vi "cwlaserShutterFromWavelength.vi"(0 "wavelength (nm)":dbl) -> (1 "shutter":i32, 2 "found":bool)   [LabVIEW 2017]
uses:
  globalDevices.vi
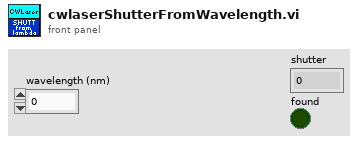
[diagram p1: front panel]
types:
  T1 = cluster{"serialPort":refnum<visa-resource-name>, "error":errorcluster, "power (mW)":dbl, "wavelength (nm)":dbl, "type":string, "shutter":i32}[]
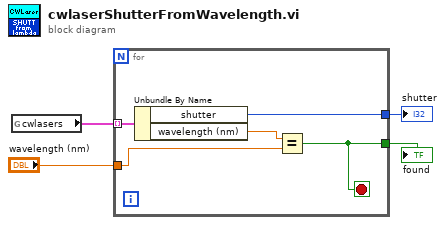
[diagram p0: block diagram]
diagram:
  n1 = global read "globalDevices.vi" "cwlasers"() -> (w4:T1)
  n2 = for {
    tunnel: w4 -> [w9] mode=indexing
    tunnel: "wavelength (nm)" -> [w7]
    tunnel: [w6] -> w2
    tunnel: [w5] -> w1
    stop <- w5 stop-if-true
    n3 = Unbundle By Name(w9) -> ("shutter"=w6:i32, "wavelength (nm)"=w8:dbl)
    n4 = Equal?(x=w8, y=w7) -> (x = y?=w5:bool)
  }
  "shutter" <- w2
  "found" <- w1
